vi "Tab Control - Colors.vi"(8 "error in (no error)":errorcluster, 10 "ctrl ref in":refnum<vi>, 11 "Material-Scheme in":refnum<class "Material-Scheme.lvclass">) -> (0 "error out":errorcluster)   [LabVIEW 2021, in "TSC Material Theme.lvlib" / "Material-Scheme.lvclass"]
doc: "Apply Color Rules to the tab control based on the tag data or defaults.\n\n<b>Code Developed By:</b>\nDaniel Coons\nTechnology Service Corporation\nwww.tsc.com/atcs"
uses:
  Material-Scheme.lvclass
  Material-Scheme.lvclass/Material-Scheme.ctl
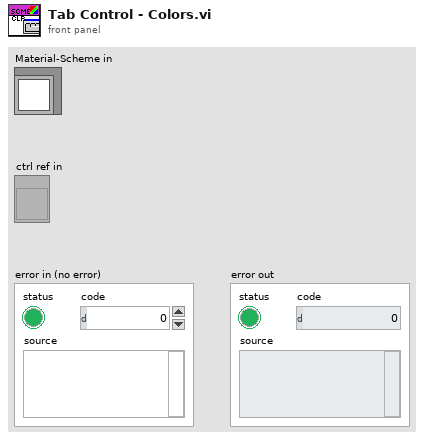
[diagram p1: front panel]
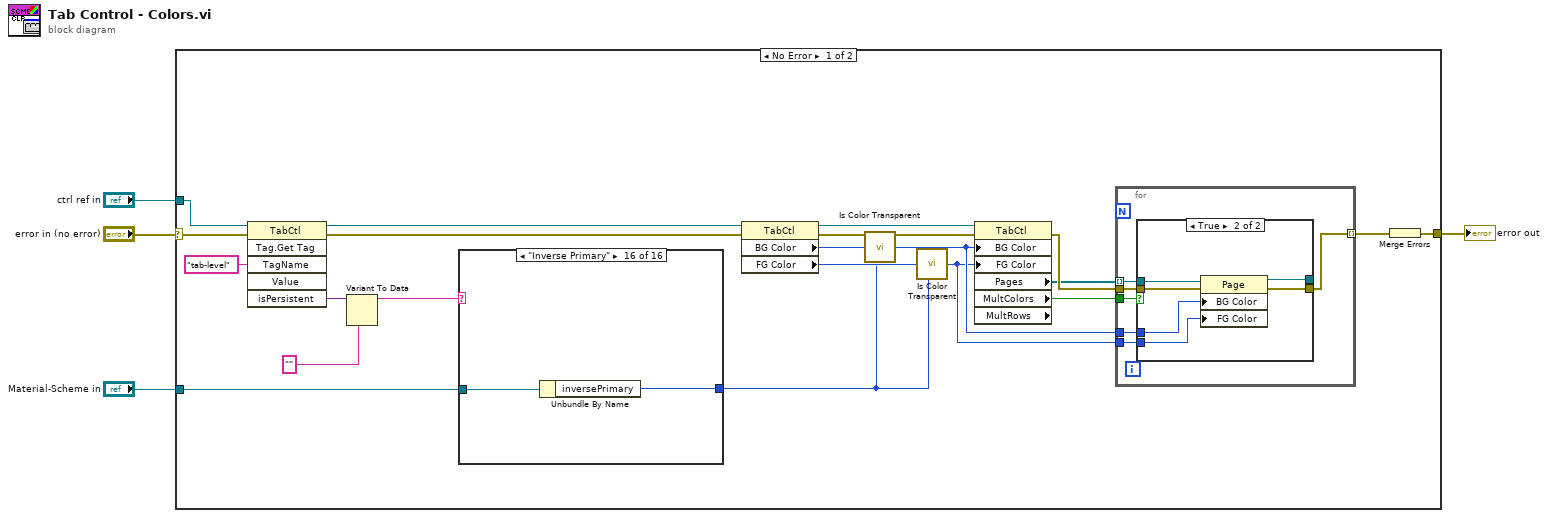
[diagram p0: block diagram]
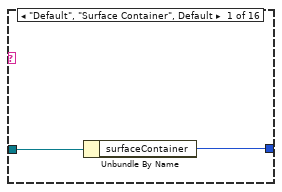
[diagram p3: hidden frame]
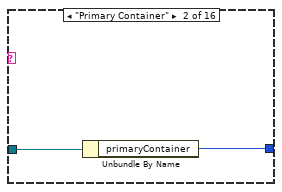
[diagram p4: hidden frame]
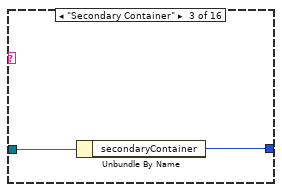
[diagram p5: hidden frame]
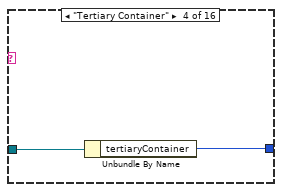
[diagram p6: hidden frame]
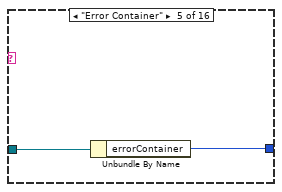
[diagram p7: hidden frame]
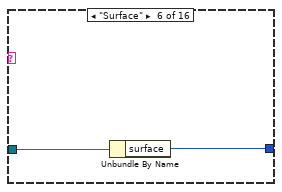
[diagram p8: hidden frame]
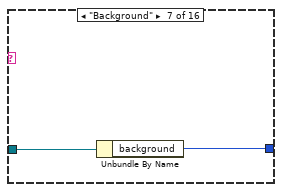
[diagram p9: hidden frame]
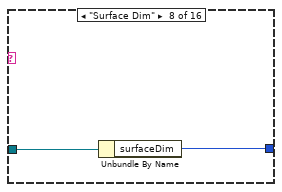
[diagram p10: hidden frame]
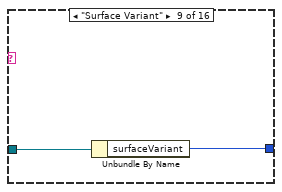
[diagram p11: hidden frame]
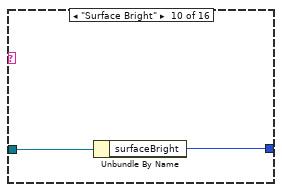
[diagram p12: hidden frame]
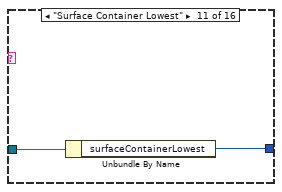
[diagram p13: hidden frame]
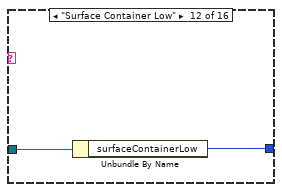
[diagram p14: hidden frame]
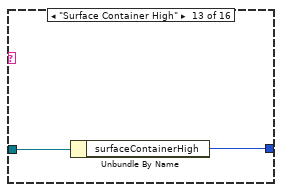
[diagram p15: hidden frame]
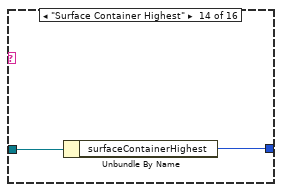
[diagram p16: hidden frame]
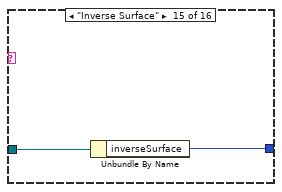
[diagram p17: hidden frame]
diagram:
  n1 = case shown="No Error" "error in (no error)" {
    selector: "error in (no error)" -> [w14 w72]
    tunnel: "Material-Scheme in" -> [w6 _]
    tunnel: [w17 w72] -> w3
    tunnel: "ctrl ref in" -> [w12 _]
    frame No Error {
      n2 = invoke class="TabCtl" method="Tag.Get Tag"(reference=w12, error in=w14, "TagName"="tab-level" ("Tag Name")) -> (reference out=w11:refnum<vi>, error out=w13:errorcluster, "isPersistent"=w9:variant)  [unwired: 3 in, 3 out]
      n3 = Variant To Data(type="", Variant=w9) -> (data=w7:string)  [unwired: 1 in, 1 out]
      n4 = case shown="\"Inverse Primary\"" w7 {
        tunnel: [w41 w43 w45 w47 w49 w51 w53 w55 w57 w59 w61 w63 w65 w67 w69 w71] -> w5
        tunnel: w6 -> [w40 w42 w44 w46 w48 w50 w52 w54 w56 w58 w60 w62 w64 w66 w68 w70]
        frame "Default", "Surface Container", Default {
          n5 = Unbundle By Name(w40) -> ("surfaceContainer"=w41:u32)
        }
        frame "Primary Container" {
          n6 = Unbundle By Name(w42) -> ("primaryContainer"=w43:u32)
        }
        frame "Secondary Container" {
          n7 = Unbundle By Name(w44) -> ("secondaryContainer"=w45:u32)
        }
        frame "Tertiary Container" {
          n8 = Unbundle By Name(w46) -> ("tertiaryContainer"=w47:u32)
        }
        frame "Error Container" {
          n9 = Unbundle By Name(w48) -> ("errorContainer"=w49:u32)
        }
        frame "Surface" {
          n10 = Unbundle By Name(w50) -> ("surface"=w51:u32)
        }
        frame "Background" {
          n11 = Unbundle By Name(w52) -> ("background"=w53:u32)
        }
        frame "Surface Dim" {
          n12 = Unbundle By Name(w54) -> ("surfaceDim"=w55:u32)
        }
        frame "Surface Variant" {
          n13 = Unbundle By Name(w56) -> ("surfaceVariant"=w57:u32)
        }
        frame "Surface Bright" {
          n14 = Unbundle By Name(w58) -> ("surfaceBright"=w59:u32)
        }
        frame "Surface Container Lowest" {
          n15 = Unbundle By Name(w60) -> ("surfaceContainerLowest"=w61:u32)
        }
        frame "Surface Container Low" {
          n16 = Unbundle By Name(w62) -> ("surfaceContainerLow"=w63:u32)
        }
        frame "Surface Container High" {
          n17 = Unbundle By Name(w64) -> ("surfaceContainerHigh"=w65:u32)
        }
        frame "Surface Container Highest" {
          n18 = Unbundle By Name(w66) -> ("surfaceContainerHighest"=w67:u32)
        }
        frame "Inverse Surface" {
          n19 = Unbundle By Name(w68) -> ("inverseSurface"=w69:u32)
        }
        frame "Inverse Primary" {
          n20 = Unbundle By Name(w70) -> ("inversePrimary"=w71:u32)
        }
      }
      n21 = property class="TabCtl"(reference=w11, error in=w13) -> (reference out=w19:refnum<vi>, error out=w18:errorcluster, "BG Color"=w20:u32, "FG Color"=w21:u32)
      n22 = call "Is Color Transparent.vi"("original color"=w20, "desired color"=w5) -> ("updated color"=w25:u32)  [unwired: 3 in]
      n23 = call "Is Color Transparent.vi"("original color"=w21, "desired color"=w5) -> ("updated color"=w24:u32)  [unwired: 3 in]
      n24 = property class="TabCtl" props=["BG Color", "FG Color", "Pages", "MultColors", "MultRows"](reference=w19, error in=w18, "BG Color"=w25, "FG Color"=w24) -> (error out=w22:errorcluster, "Pages"=w15:refnum<vi>[], "MultColors"=w23:bool)  [unwired: 2 out]
      n25 = for {
        tunnel: w22 -> [w30]
        tunnel: w15 -> [w29] mode=indexing
        tunnel: [w31] -> w16 mode=indexing
        tunnel: w23 -> [w28]
        tunnel: w24 -> [w27]
        tunnel: w25 -> [w26]
        n26 = case shown="True" w28 {
          tunnel: w30 -> [w32 w39]
          tunnel: w29 -> [w33 w38]
          tunnel: [w32 w37] -> w31
          tunnel: [w33 w36] -> _
          tunnel: w27 -> [_ w35]
          tunnel: w26 -> [_ w34]
          frame False {
          }
          frame True {
            n27 = property class="Page"(reference=w38, error in=w39, "BG Color"=w34, "FG Color"=w35) -> (reference out=w36:refnum<vi>, error out=w37:errorcluster)
          }
        }
      }
      n28 = Merge Errors(w16) -> (w17:errorcluster)
    }
    frame Error {
    }
  }
  "error out" <- w3
